vi "Optomize Settings.vi"(5 "Aviod Zone":cluster{"pos 1":dbl, "pos 2":dbl} {"pos 1" format="%#.3g"; "pos 2" format="%#.3g"}, 7 "Previous Swerve Setting":T1 {"Back Right"."Angle" scale format="%.3f"; "Back Right"."Velocity" scale=-1.0..1.0 scale format="%.1f"; "Back Left"."Angle" scale format="%.3f"; "Back Left"."Velocity" scale=-1.0..1.0 scale format="%.1f"; "Front Left"."Angle" scale format="%.3f"; "Front Left"."Velocity" scale=-1.0..1.0 scale format="%.1f"; "Front Right"."Angle" scale format="%.3f"; "Front Right"."Velocity" scale=-1.0..1.0 scale format="%.1f"}, 11 "Swerve Request":T1 {"Back Right"."Angle" scale format="%.3f"; "Back Right"."Velocity" scale=-1.0..1.0 scale format="%.1f"; "Back Left"."Angle" scale format="%.3f"; "Back Left"."Velocity" scale=-1.0..1.0 scale format="%.1f"; "Front Left"."Angle" scale format="%.3f"; "Front Left"."Velocity" scale=-1.0..1.0 scale format="%.1f"; "Front Right"."Angle" scale format="%.3f"; "Front Right"."Velocity" scale=-1.0..1.0 scale format="%.1f"}) -> (3 "Swerve Setting Out":T1 {"Back Right"."Angle" scale format="%.3f"; "Back Right"."Velocity" scale=-1.0..1.0 scale format="%.1f"; "Back Left"."Angle" scale format="%.3f"; "Back Left"."Velocity" scale=-1.0..1.0 scale format="%.1f"; "Front Left"."Angle" scale format="%.3f"; "Front Left"."Velocity" scale=-1.0..1.0 scale format="%.1f"; "Front Right"."Angle" scale format="%.3f"; "Front Right"."Velocity" scale=-1.0..1.0 scale format="%.1f"})   [LabVIEW 2023, in "Thor-SwerveDrive_ACT.lvlib"]
uses:
  Thor-SwerveDrive_ACT.lvlib
  Shared Code/TypeDefs/Level_Velocity plus-minus 1.ctl
  Shared Code/TypeDefs/Dial_Compase heading unit circle CCW positive.ctl
  Shared Code/TypeDefs/Cluster_Module Velocity-Direction-Rotations.ctl
  Shared Code/TypeDefs/Cluster_Swerve 4 Steer and Velocity.ctl
panel:
  # "\"Front\" of Robot"
  # "Right Hand Rule"
  # "X"
  # "+CCW"
  # "Y"
  # "(0,0)"
  # "\"Front\" of Robot"
  # "Right Hand Rule"
  # "X"
  # "+CCW"
  # "Y"
  # "(0,0)"
  # "\"Front\" of Robot"
  # "Right Hand Rule"
  # "X"
  # "+CCW"
  # "Y"
  # "(0,0)"
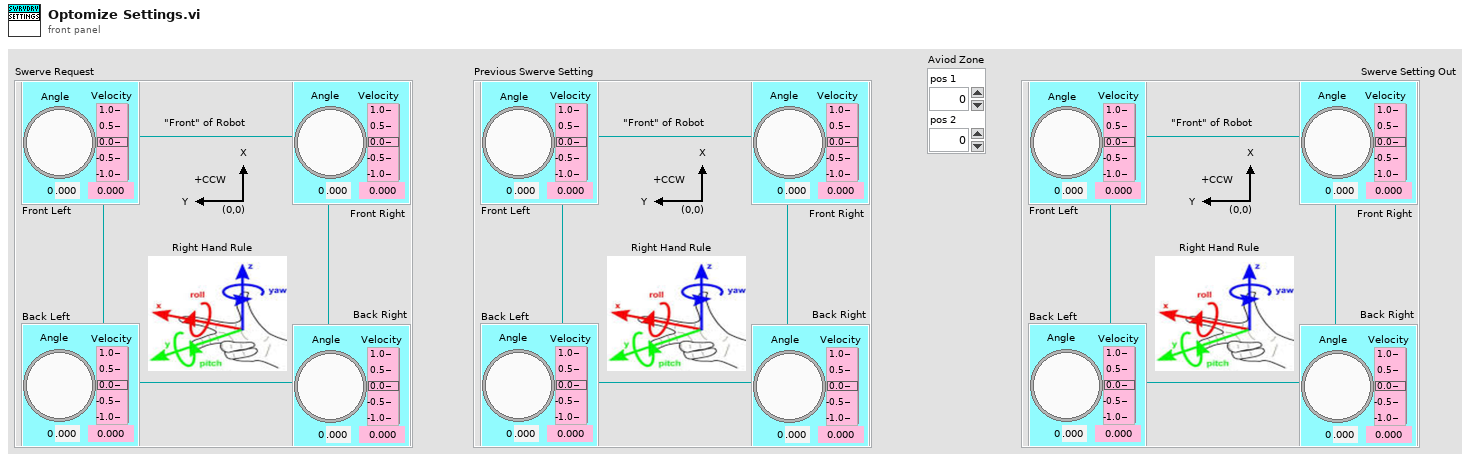
[diagram p1: front panel]
types:
  T1 = typedef "Cluster_Swerve 4 Steer and Velocity.ctl" = cluster{"Front Right":T2, "Front Left":T2, "Back Left":T2, "Back Right":T2}
  T2 = typedef "Cluster_Module Velocity-Direction-Rotations.ctl" = cluster{"Velocity":T3, "Angle":T4, "Rotations Count":dbl}
  T3 = typedef "Level_Velocity plus-minus 1.ctl" = dbl
  T4 = typedef "Dial_Compase heading unit circle CCW positive.ctl" = dbl
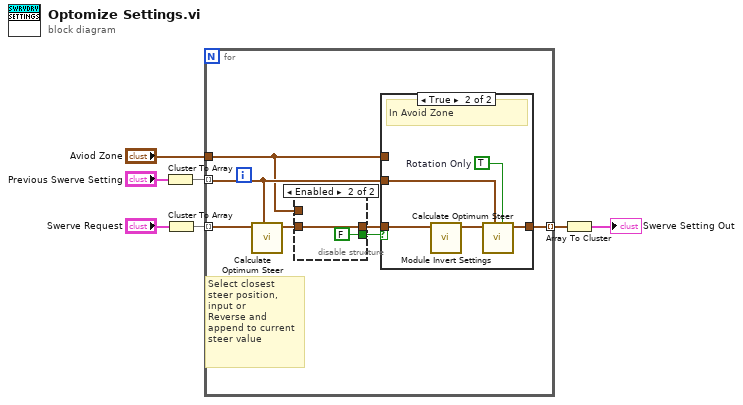
[diagram p0: block diagram]
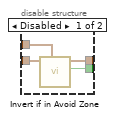
[diagram p2: hidden frame]
diagram:
  n1 = Cluster To Array(cluster="Previous Swerve Setting") -> (array=w3:T2[])
  n2 = Cluster To Array(cluster="Swerve Request") -> (array=w5:T2[])
  n3 = for {
    tunnel: w5 -> [w10] mode=indexing
    tunnel: "Aviod Zone" -> [w8]
    tunnel: w3 -> [w12] mode=indexing
    tunnel: [w11] -> w2 mode=indexing
    # "Select closest\nsteer position,\ninput or\nReverse and\nappend to current\nsteer value"
    n4 = call "Calculate Optimum Steer.vi"("Previous Set Swerve"=w12, "New Swerve"=w10) -> ("Set Swerve Out"=w14:T2)  [unwired: 9 in]
    n5 = disable-structure shown="Enabled" {
      disable-tunnel: w14 -> [w18 w20]
      disable-tunnel: [w17 FALSE ("In Avoid Zone")] -> w13
      disable-tunnel: [w16 w20] -> w9
      disable-tunnel: w8 -> [w15 _]
      frame Disabled {
        n6 = call "Invert if in Avoid Zone.vi"("Avoid Zone (Unit Circle)"=w15, "Set Values"=w18) -> ("In Avoid Zone"=w17:bool, "Set Values Out"=w16:T2)  [unwired: 8 in]
      }
      frame Enabled {
      }
    }
    n7 = case shown="True" w13 {
      tunnel: w8 -> [_ _]
      tunnel: w12 -> [_ w26]
      tunnel: [w21 w25] -> w11
      tunnel: w9 -> [w21 w23]
      frame False {
        # "Not in Avoid Zone"
      }
      frame True {
        w22 = TRUE  # Rotation Only
        # "In Avoid Zone"
        n8 = call "Module Invert Settings.vi"("Setting"=w23) -> ("Inverted Setting Out"=w24:T2)  [unwired: 10 in]
        n9 = call "Calculate Optimum Steer.vi"("Rotation Only"=w22, "Previous Set Swerve"=w26, "New Swerve"=w24) -> ("Set Swerve Out"=w25:T2)  [unwired: 8 in]
      }
    }
  }
  n10 = Array To Cluster(array=w2) -> (cluster=→"Swerve Setting Out":cluster{"[0]":T2, "[1]":T2, "[2]":T2, "[3]":T2})
